vi "LoadMainPanel.vi"(8 "error in (no error)":errorcluster, 11 "MPC_AutoPast in":refnum<class "MPC_AutoInspection.lvclass">) -> (0 "error out":errorcluster, 2 "This VI":refnum<vi>, 3 "MPC_AutoPast out":refnum<class "MPC_AutoInspection.lvclass">)   [LabVIEW 2019, in "MPC_AutoInspection.lvclass"]
uses:
  MPC_AutoInspection.lvclass
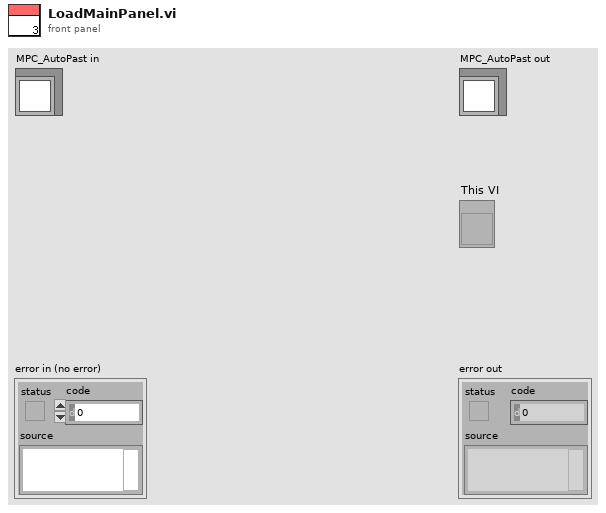
[diagram p1: front panel]
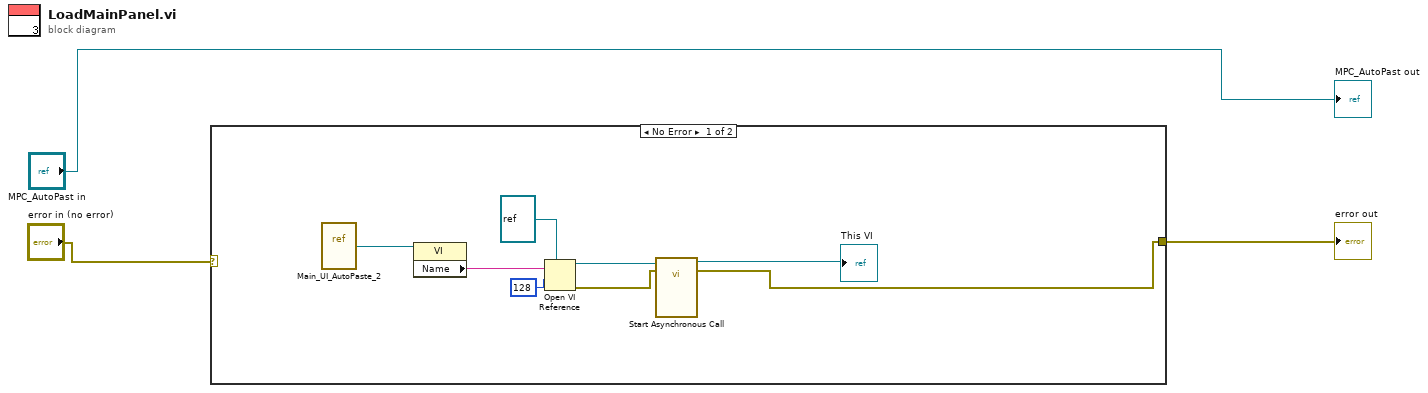
[diagram p0: block diagram]
diagram:
  n1 = case shown="No Error" "error in (no error)" {
    selector: "error in (no error)" -> [_ w12]
    tunnel: [w5 w12] -> w1
    frame No Error {
      n2 = vi-ref "Main_UI_AutoPaste_2.vi"() -> (w8:refnum<vi>)
      n3 = property class="VI"(reference=w8) -> ("Name"=w7:string)  [unwired: 1 in, 2 out]
      n4 = Open VI Reference(type specifier VI Refnum (for type only)=refnum<vi> refnum, vi path=w7, options=128) -> (vi reference=w11:refnum<vi>, error out=w4:errorcluster)  [unwired: 3 in]
      n5 = call-by-ref "Start Asynchronous Call"(reference=w11, error in=w4) -> (reference out=→"This VI":refnum<vi>, error out=w5:errorcluster)  [unwired: 11 in, 1 out]
    }
    frame Error {
    }
  }
  "error out" <- w1
  "MPC_AutoPast out" <- "MPC_AutoPast in"
